vi "SetTimesliceDialog.vi"(11 "timeslice in":T1) -> (3 "timeslice out":T1)   [LabVIEW 2014]
uses:
  controls/Timeslice.ctl
panel:
  in  "Duration":dbl[](array[numeric])
  in  "names":string[](array[string])
  out "size(s) 2":i32[](array[numeric])
  in  "TS":bool[][](array[boolean])
  in  "Cancel Button":bool
  in  "OK Button":bool
  in  "error in (no error)":errorcluster
  out "error out":errorcluster
  out "UI Refresh Needed?":bool
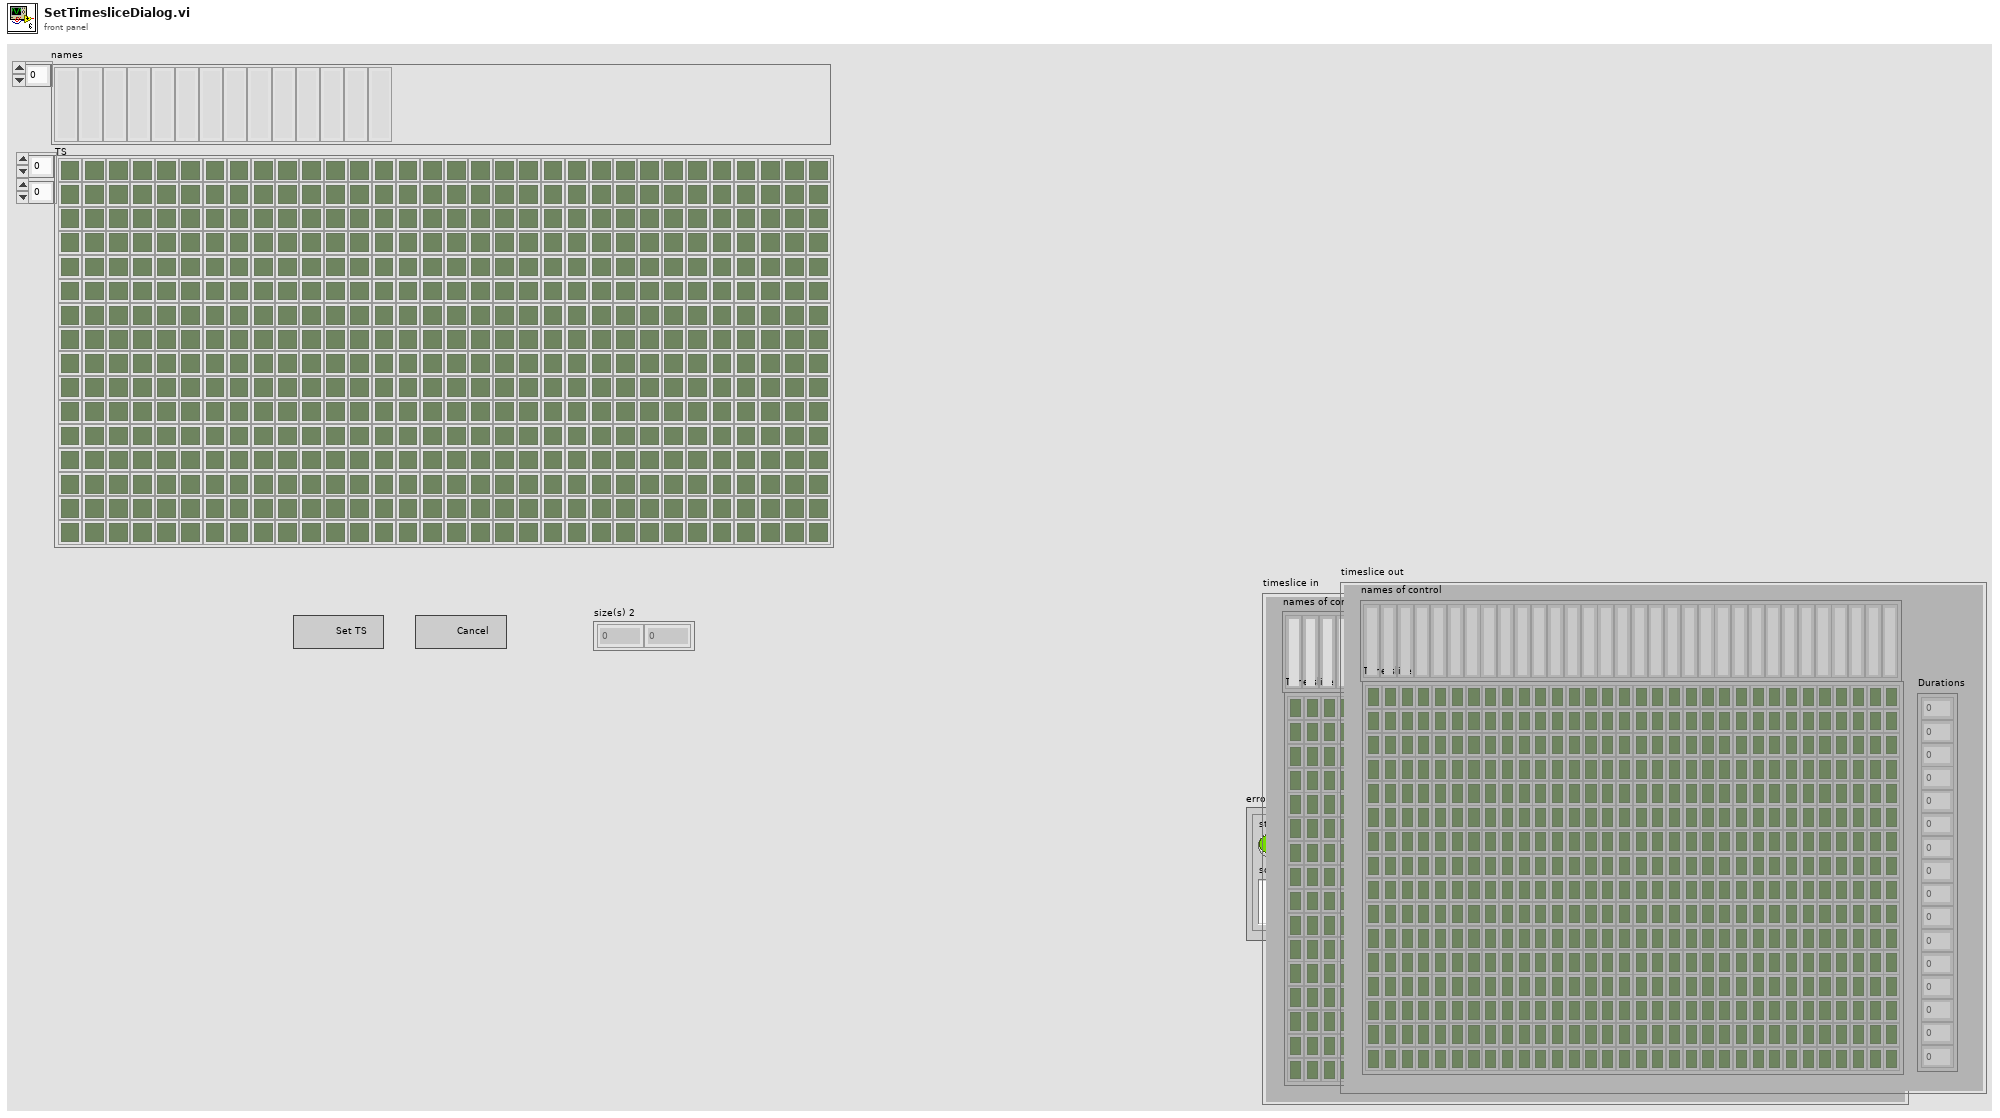
[diagram p1: front panel]
types:
  T1 = typedef "Timeslice.ctl" = cluster{"Time slice":bool[][], "Durations":dbl[], "names of control":string[]}
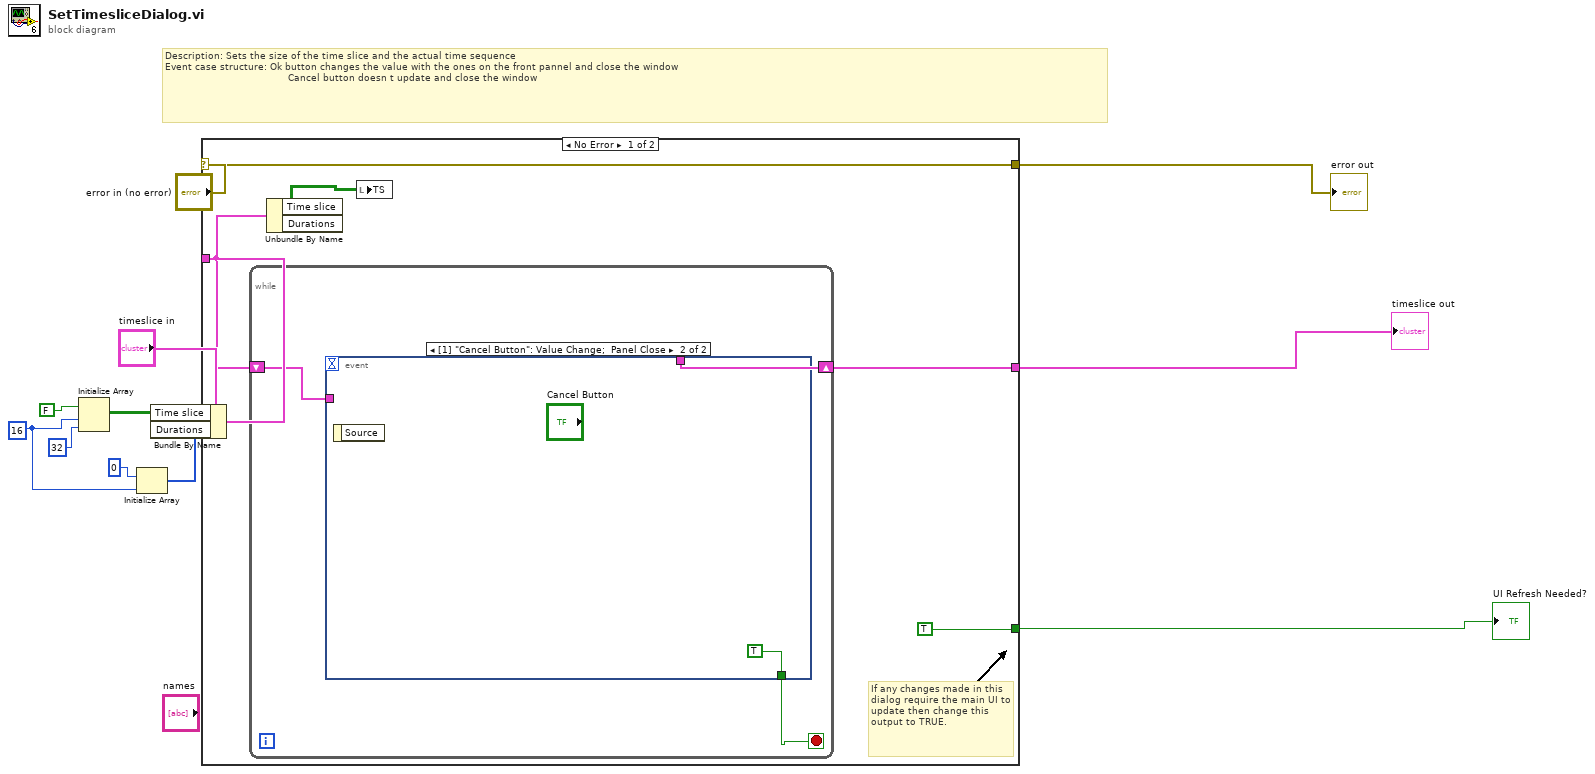
[diagram p0: block diagram]
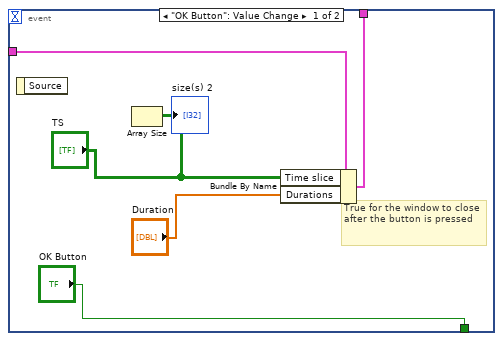
[diagram p2: hidden frame]
diagram:
  w3 = 16
  # "Description: Sets the size of the time slice and the actual time sequence\nEvent case structure: Ok button changes the value with the ones on the front pannel and close the window\n                                         Cancel button doesn t update and close the window"
  n1 = Initialize Array(FALSE, w3, 32) -> (w6:bool[][])
  n2 = Initialize Array(0, w3) -> (w1:i32[])
  n3 = Bundle By Name(cluster="timeslice in", "Time slice"=w6, "Durations"=w1) -> (w4:T1)
  n4 = case shown="No Error" "error in (no error)" {
    selector: "error in (no error)" -> [w16 w29]
    tunnel: [w16 w29] -> w11
    tunnel: [w15 w28] -> w9
    tunnel: [TRUE ("UI Refresh Needed?") _] -> w10
    tunnel: w4 -> [w13 w28]
    frame No Error {
      # "If any changes made in this dialog require the main UI to update then change this output to TRUE."
      n5 = while {
        shift-right: [w19] -> w15
        shift-left: w13 -> [w20]
        stop <- w18 stop-if-true
        n6 = event shown="[1] \"Cancel Button\": Value Change;  Panel Close" {
          selector: _ -> [_ _]
          dyn-events: _ -> [_ _]
          timeout: _ -> [_ _]
          tunnel: ["OK Button" TRUE] -> w18
          tunnel: w20 -> [w26 _]
          tunnel: [w25 _] -> w19
          event "OK Button": Value Change {
            # "True for the window to close after the button is pressed"
            n7 = event-data() -> ()  [unwired: 1 in, 1 out]
            n8 = Array Size(array="TS") -> (size(s)=→"size(s) 2":i32[])
            n9 = Bundle By Name(cluster=w26, "Time slice"="TS", "Durations"="Duration") -> (w25:T1)
          }
          event "Cancel Button": Value Change; Panel Close {
            n10 = event-data() -> ()  [unwired: 1 in, 1 out]
          }
        }
      }
      n11 = Unbundle By Name(w13) -> ("Time slice"=w14:bool[][])  [unwired: 1 out]
      n12 = local write "TS"(w14) -> ()
    }
    frame Error {
    }
  }
  "UI Refresh Needed?" <- w10
  "error out" <- w11
  "timeslice out" <- w9
